vi "NIIE_MouseDown.vi"(7 "Flip Colors?":bool, 8 "Error":errorcluster, 10 "Coords":T5, 11 "Data":T1={"Class"={"Ants"=refnum, "Layer"=refnum, "Templates"=refnum, "Icon"=refnum, "Glyph"=refnum, "Settings"=refnum, "Tools"=refnum}, "Ref"={"Add Layer"=refnum, "Remove Layer"=refnum, "Line Text"=[], "Body Text Spec"=refnum, "DNL_Font"=refnum, "glyph path str"=refnum, "templates path str"=refnum, "Arrow Up"=refnum, "Arrow Down"=refnum, "IE VI Ref"=refnum, "Glyphs tree"=refnum, "Templates tree"=refnum, "Layer Icon Text"=refnum, "Layer Template"=refnum, "Clipboard"=refnum, "BW icon in"=refnum, "Color icon in"=refnum, "Layer Clust"=refnum, "Body Text"=refnum, "DNL_Framework Templates"=refnum, "Search Templates"=refnum, "TextMarker"=refnum, "Tab Control"=refnum, "Search Glyphs"=refnum, "Line Color"=refnum, "DNL_Glyphs []"=refnum, "Fill Color"=refnum, "Tools"=refnum, "Glyphs tree"=refnum, "Icon"=refnum, "Preview"=refnum, "Ants"=refnum, "Terminals"=refnum, "menu reference"=refnum, "LayerNames"=[], "GlyphLoadAnimation"=refnum, "TemplateLoadAnimation"=refnum, "refreshGlyphs"=refnum, "refreshTemplates"=refnum}, "Support"={"AntsRect"={"left"=0, "top"=0, "right"=0, "bottom"=0}, "Mouse Move Coords"={"Horizontal"=0, "Vertical"=0}, "Mouse Down Coords"={"Horizontal"=0, "Vertical"=0}, "Temp Coord"={"Horizontal"=0, "Vertical"=0}, "Action"=enum."Default", "Edge Color"=4914962, "Fill Color"=16860, "Mouse Down?"=FALSE, "Draft Mode?"=FALSE, "Temp Icon"=bytes[3102], "CTRL Pressed"=FALSE, "Move Selection?"=FALSE, "AntsRect Orig"={"left"=0, "top"=0, "right"=0, "bottom"=0}, "Text"="", "TM Set?"=FALSE, "Mouse inside icon?"=FALSE, "Tool (old value)"=0, "Pencil Move Color"=0, "Swap Colors?"=FALSE, "Shift pressed?"=FALSE}}) -> (0 "Error Out":errorcluster, 3 "Data Out":T1={"Class"={"Ants"=refnum, "Layer"=refnum, "Templates"=refnum, "Icon"=refnum, "Glyph"=refnum, "Settings"=refnum, "Tools"=refnum}, "Ref"={"Add Layer"=refnum, "Remove Layer"=refnum, "Line Text"=[], "Body Text Spec"=refnum, "DNL_Font"=refnum, "glyph path str"=refnum, "templates path str"=refnum, "Arrow Up"=refnum, "Arrow Down"=refnum, "IE VI Ref"=refnum, "Glyphs tree"=refnum, "Templates tree"=refnum, "Layer Icon Text"=refnum, "Layer Template"=refnum, "Clipboard"=refnum, "BW icon in"=refnum, "Color icon in"=refnum, "Layer Clust"=refnum, "Body Text"=refnum, "DNL_Framework Templates"=refnum, "Search Templates"=refnum, "TextMarker"=refnum, "Tab Control"=refnum, "Search Glyphs"=refnum, "Line Color"=refnum, "DNL_Glyphs []"=refnum, "Fill Color"=refnum, "Tools"=refnum, "Glyphs tree"=refnum, "Icon"=refnum, "Preview"=refnum, "Ants"=refnum, "Terminals"=refnum, "menu reference"=refnum, "LayerNames"=[], "GlyphLoadAnimation"=refnum, "TemplateLoadAnimation"=refnum, "refreshGlyphs"=refnum, "refreshTemplates"=refnum}, "Support"={"AntsRect"={"left"=0, "top"=0, "right"=0, "bottom"=0}, "Mouse Move Coords"={"Horizontal"=0, "Vertical"=0}, "Mouse Down Coords"={"Horizontal"=0, "Vertical"=0}, "Temp Coord"={"Horizontal"=0, "Vertical"=0}, "Action"=enum."Default", "Edge Color"=4914962, "Fill Color"=16860, "Mouse Down?"=FALSE, "Draft Mode?"=FALSE, "Temp Icon"=bytes[3102], "CTRL Pressed"=FALSE, "Move Selection?"=FALSE, "AntsRect Orig"={"left"=0, "top"=0, "right"=0, "bottom"=0}, "Text"="", "TM Set?"=FALSE, "Mouse inside icon?"=FALSE, "Tool (old value)"=0, "Pencil Move Color"=0, "Swap Colors?"=FALSE, "Shift pressed?"=FALSE}})   [LabVIEW 2021]
uses:
  <vilib>/Utility/miscctls.llb/LVPoint32TypeDef.ctl
  Controls/IE Data.ctl
  Class/Ants/Ants.lvclass
  Class/FakedArray/FakedArray.lvclass
  Class/Icon Library/Glyph.lvclass
  Class/Settings/Settings.lvclass
  Class/Tools/Tools Paint.lvclass
  vi.lib/LabVIEW Icon API/lv_icon/Classes/Icon/Icon.lvclass
  Controls/IE Classes.ctl
  Controls/References Cluster.ctl
  Controls/SupportClass.ctl
  Controls/ENUM_SupportClass_Action.ctl
  vi.lib/LabVIEW Icon API/lv_icon/Controls/IEColor.ctl
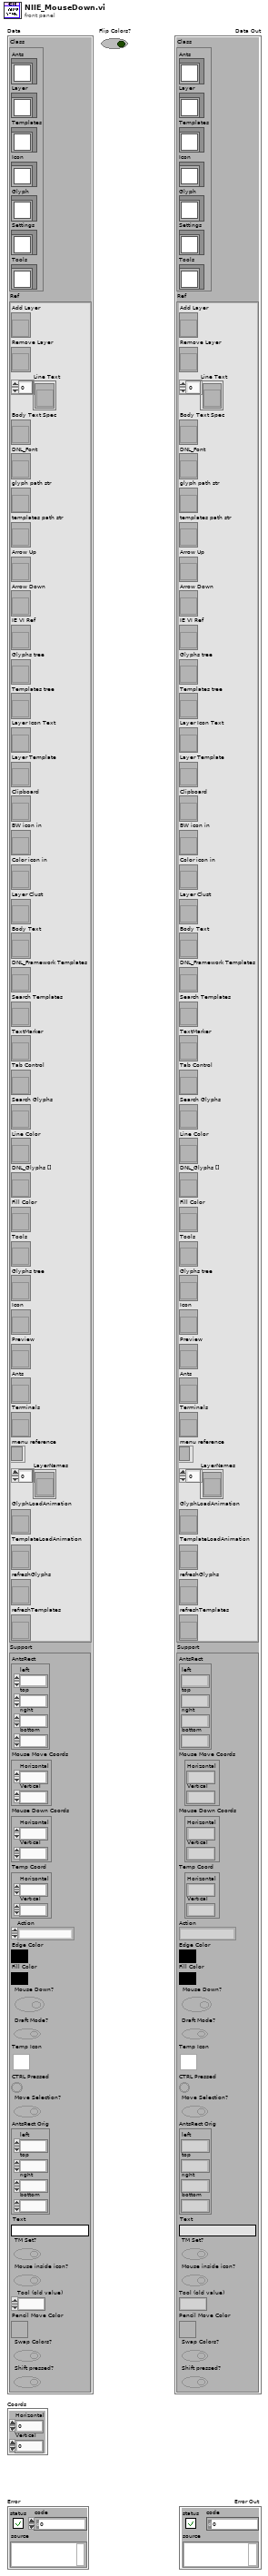
[diagram p1: front panel]
types:
  T1 = typedef "IE Data.ctl" = cluster{"Class":T2, "Ref":T3, "Support":T4}
  T2 = typedef "IE Classes.ctl" = cluster{"Ants":refnum<class "Ants.lvclass">, "Layer":refnum<class "FakedArray.lvclass">, "Templates":refnum<class "FakedArray.lvclass">, "Icon":refnum<class "Icon.lvclass">, "Glyph":refnum<class "Glyph.lvclass">, "Settings":refnum<class "Settings.lvclass">, "Tools":refnum<class "Tools Paint.lvclass">}
  T3 = typedef "References Cluster.ctl" = cluster{"Add Layer":refnum<vi>, "Remove Layer":refnum<vi>, "Line Text":refnum<vi>[], "Body Text Spec":refnum<vi>, "DNL_Font":refnum<vi>, "glyph path str":refnum<vi>, "templates path str":refnum<vi>, "Arrow Up":refnum<vi>, "Arrow Down":refnum<vi>, "IE VI Ref":refnum<vi>, "Glyphs tree":refnum<vi>, "Templates tree":refnum<vi>, "Layer Icon Text":refnum<vi>, "Layer Template":refnum<vi>, "Clipboard":refnum<vi>, "BW icon in":refnum<vi>, "Color icon in":refnum<vi>, "Layer Clust":refnum<vi>, "Body Text":refnum<vi>, "DNL_Framework Templates":refnum<vi>, "Search Templates":refnum<vi>, "TextMarker":refnum<vi>, "Tab Control":refnum<vi>, "Search Glyphs":refnum<vi>, "Line Color":refnum<vi>, "DNL_Glyphs []":refnum<vi>, "Fill Color":refnum<vi>, "Tools":refnum<vi>, "Glyphs tree":refnum<vi>, "Icon":refnum<vi>, "Preview":refnum<vi>, "Ants":refnum<vi>, "Terminals":refnum<vi>, "menu reference":refnum<k9>, "LayerNames":refnum<vi>[], "GlyphLoadAnimation":refnum<vi>, "TemplateLoadAnimation":refnum<vi>, "refreshGlyphs":refnum<vi>, "refreshTemplates":refnum<vi>}
  T4 = typedef "SupportClass.ctl" = cluster{"AntsRect":cluster{"left":i16, "top":i16, "right":i16, "bottom":i16}, "Mouse Move Coords":T5, "Mouse Down Coords":T5, "Temp Coord":T5, "Action":T6, "Edge Color":T7, "Fill Color":T7, "Mouse Down?":bool, "Draft Mode?":bool, "Temp Icon":picture, "CTRL Pressed":bool, "Move Selection?":bool, "AntsRect Orig":cluster{"left":i16, "top":i16, "right":i16, "bottom":i16}, "Text":string, "TM Set?":bool, "Mouse inside icon?":bool, "Tool (old value)":u32, "Pencil Move Color":u32, "Swap Colors?":bool, "Shift pressed?":bool}
  T5 = typedef "LVPoint32TypeDef.ctl" = cluster{"Horizontal":i32, "Vertical":i32}
  T6 = typedef "ENUM_SupportClass_Action.ctl" = enum16{"Default", "Move Selection", "Glyph Library", "Tool"}
  T7 = typedef "IEColor.ctl" = u32
  T8 = cluster{"left":i16, "top":i16, "right":i16, "bottom":i16}
  T9 = typedef "Cluster_Button Draw Tools.ctl" = enum32{"Pencil", "Line", "Dropper", "Fill", "Rectangle", "Filled Rectangle", "Ellipse", "Filled Ellipse", "Eraser", "Text", "Select", "Move"}
  T10 = cluster{"Horizontal":i32, "Vertical":i32, "Vertical 2":i32, "Vertical 3":i32}
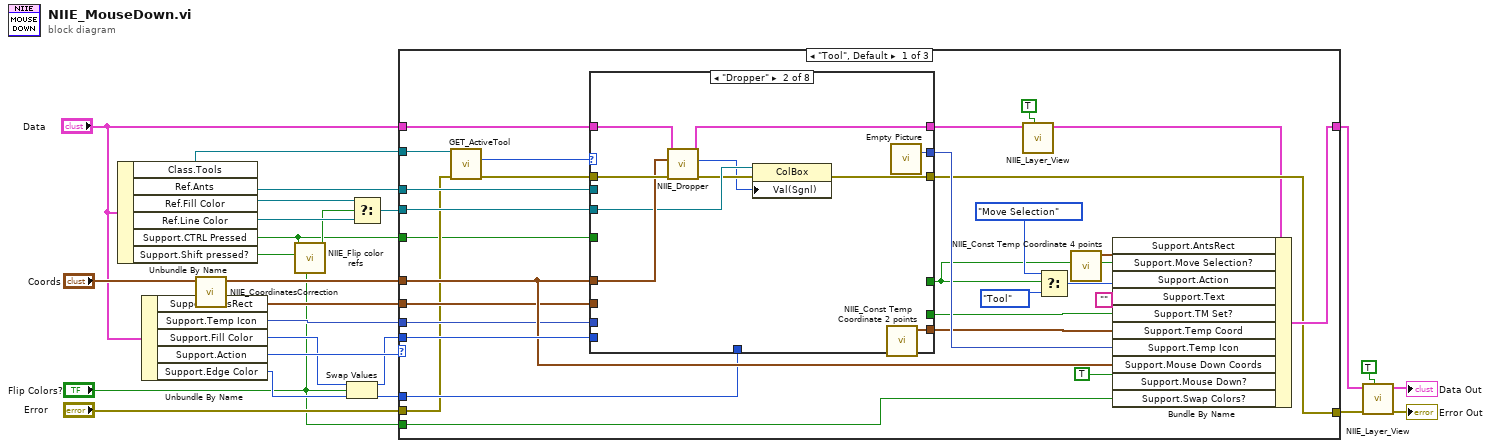
[diagram p0: block diagram]
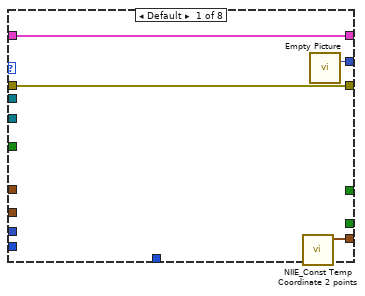
[diagram p2: hidden frame]
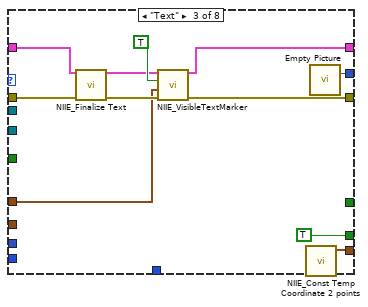
[diagram p3: hidden frame]
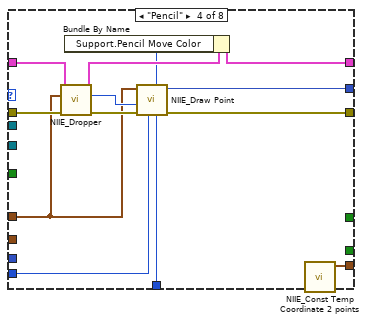
[diagram p4: hidden frame]
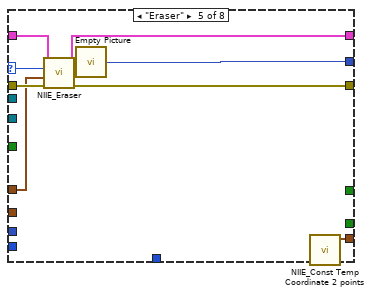
[diagram p5: hidden frame]
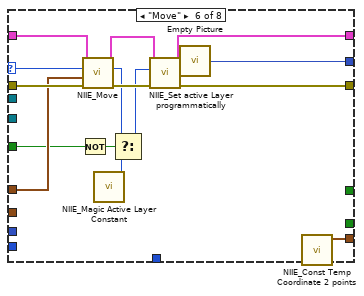
[diagram p6: hidden frame]
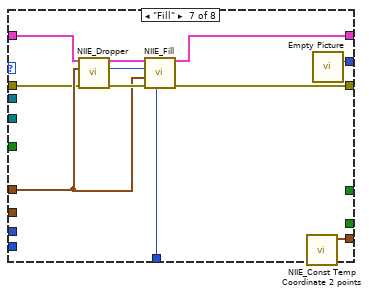
[diagram p7: hidden frame]
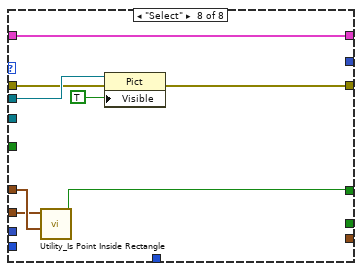
[diagram p8: hidden frame]
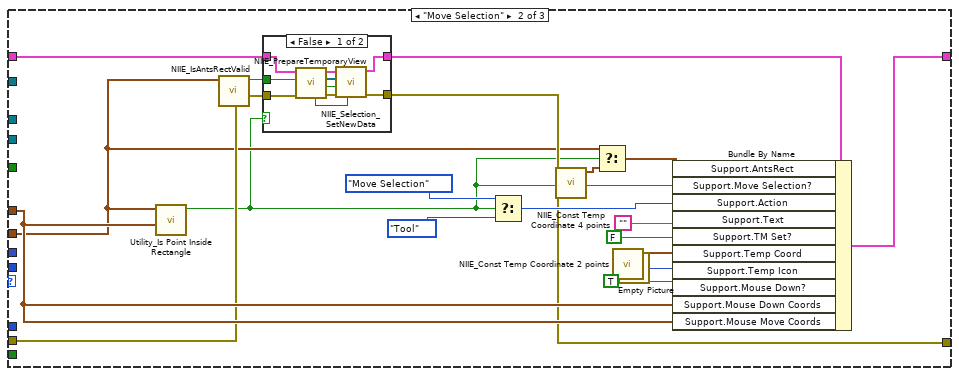
[diagram p9: hidden frame]
diagram:
  n1 = Unbundle By Name("Data") -> ("Class.Tools"=w19:refnum<class "Tools Paint.lvclass">, "Ref.Ants"=w21:refnum<vi>, "Ref.Fill Color"=w6:refnum<vi>, "Ref.Line Color"=w5:refnum<vi>, "Support.CTRL Pressed"=w1:bool, "Support.Shift pressed?"=w2:bool)
  n2 = Unbundle By Name("Data") -> ("Support.AntsRect"=w20:T8, "Support.Temp Icon"=w22:picture, "Support.Fill Color"=w9:T7, "Support.Action"=w24:T6, "Support.Edge Color"=w11:T7)
  n3 = call "NIIE_CoordinatesCorrection.vi"("Coordinates In"="Coords") -> ("Corrected Out"=w25:T5)  [unwired: 10 out]
  n4 = call "NIIE_Flip color refs.vi"("Flip colors?"="Flip Colors?", "Shift pressed"=w2, "CTRL pressed"=w1) -> ("Flip?"=w3:bool)  [unwired: 8 out]
  n5 = Swap Values(12:w9, 13:"Flip Colors?", 14:w11) -> (1:w8:T7, 3:w10:T7)
  n6 = Select(t=w6, s=w3, f=w5) -> (s? t:f=w7:refnum<vi>)
  n7 = case shown="\"Tool\", Default" w24 {
    tunnel: [w47 w141 w167] -> w15
    tunnel: w25 -> [w50 w144 _]
    tunnel: "Error" -> [w34 w142 w167]
    tunnel: [w48 w149 w166] -> w12
    tunnel: w8 -> [w51 _ _]
    tunnel: w10 -> [w46 _ _]
    tunnel: w22 -> [w43 _ _]
    tunnel: w21 -> [w42 _ _]
    tunnel: w20 -> [w41 w138 _]
    tunnel: w7 -> [w37 _ _]
    tunnel: w19 -> [w35 _ _]
    tunnel: "Data" -> [w33 w140 w166]
    tunnel: "Flip Colors?" -> [w32 _ _]
    tunnel: w1 -> [w30 _ _]
    frame "Tool", Default {
      n8 = call-dynamic "GET_ActiveTool.vi"("error in (no error)"=w34, "Tools Paint.lvclass in"=w35) -> ("error out"=w53:errorcluster, "Radio Buttons"=w54:T9)  [unwired: 8 out]
      n9 = case shown="\"Dropper\"" w54 {
        selector: w54 -> [_ _ _ _ w96 w112 _ _]
        tunnel: w53 -> [w58 w67 w75 w90 w99 w114 w121 w129]
        tunnel: w50 -> [_ w65 w69 w81 w97 w113 w122 w131]
        tunnel: w51 -> [_ _ _ w82 _ _ _ _]
        tunnel: [w57 w68 w76 w80 w100 w115 w125 _] -> w49
        tunnel: [w58 w66 w78 w92 w98 w109 w124 w132] -> w47
        tunnel: w46 -> [_ _ _ w83 _ _ w116 _]
        tunnel: [w56 w64 w79 w91 w95 w111 w126 _] -> w45
        tunnel: [_ _ TRUE ("Mouse Down?") _ _ _ _ _] -> w44
        tunnel: w43 -> [_ _ _ _ _ _ _ _]
        tunnel: w42 -> [_ _ _ _ _ _ _ w134]
        tunnel: w41 -> [_ _ _ _ _ _ _ w130]
        tunnel: [_ _ _ _ _ _ _ w127] -> w36
        tunnel: w37 -> [_ w63 _ _ _ _ _ _]
        tunnel: w33 -> [w55 w62 w73 w87 w94 w108 w119 w128]
        tunnel: [w55 w61 w70 w85 w93 w106 w117 w128] -> w28
        tunnel: w30 -> [_ _ _ _ _ w105 _ _]
        frame Default {
          n10 = call "NIIE_Const Temp Coordinate 2 points.vi"() -> ("Const Temp Coordinate"=w56:T5)  [unwired: 11 out]
          n11 = call "Empty Picture"() -> ("empty picture"=w57:picture)
        }
        frame "Dropper" {
          n12 = call "NIIE_Dropper.vi"("Error"=w67, "Point"=w65, "Data"=w62) -> ("Error Out"=w60:errorcluster, "Color Out"=w59:u32, "Data Out"=w61:T1)  [unwired: 1 in, 5 out]
          n13 = property on="Property Node" class="ColBox"(reference=w63, error in=w60, "Val(Sgnl)"=w59) -> (error out=w66:errorcluster)  [unwired: 1 out]
          n14 = call "NIIE_Const Temp Coordinate 2 points.vi"() -> ("Const Temp Coordinate"=w64:T5)  [unwired: 11 out]
          n15 = call "Empty Picture"() -> ("empty picture"=w68:picture)
        }
        frame "Text" {
          n16 = call "NIIE_Finalize Text.vi"("Error"=w75, "Data"=w73) -> ("Error Out"=w74:errorcluster, "Data Out"=w71:T1)  [unwired: 8 out]
          n17 = call "NIIE_VisibleTextMarker.vi"("Error"=w74, "Positon"=w69, "Visible"=TRUE, "Data"=w71) -> ("Error Out"=w78:errorcluster, "Data Out"=w70:T1)  [unwired: 6 out]
          n18 = call "NIIE_Const Temp Coordinate 2 points.vi"() -> ("Const Temp Coordinate"=w79:T5)  [unwired: 11 out]
          n19 = call "Empty Picture"() -> ("empty picture"=w76:picture)
        }
        frame "Pencil" {
          n20 = call "NIIE_Dropper.vi"("Error"=w90, "Point"=w81, "Data"=w87) -> ("Error Out"=w89:errorcluster, "Color Out"=w88:u32, "Data Out"=w86:T1)  [unwired: 6 out]
          n21 = call "NIIE_Draw Point.vi"("Edge Color"=w83, "Fill Color"=w82, "Error"=w89, "Current Color (T)"=w88, "Point(x,y)"=w81) -> ("Error Out"=w92:errorcluster, "New Picture Out"=w80:picture, "Current Line Color Out"=w84:u32)  [unwired: 4 in]
          n22 = Bundle By Name(cluster=w86, "Support.Pencil Move Color"=w84) -> (w85:T1)
          n23 = call "NIIE_Const Temp Coordinate 2 points.vi"() -> ("Const Temp Coordinate"=w91:T5)  [unwired: 11 out]
        }
        frame "Eraser" {
          n24 = call "NIIE_Eraser.vi"("Error"=w99, "Point Out"=w97, "Radio Buttons"=w96, "Data"=w94) -> ("Error Out"=w98:errorcluster, "Data Out"=w93:T1)  [unwired: 1 in, 5 out]
          n25 = call "Empty Picture"() -> ("empty picture"=w100:picture)
          n26 = call "NIIE_Const Temp Coordinate 2 points.vi"() -> ("Const Temp Coordinate"=w95:T5)  [unwired: 11 out]
        }
        frame "Move" {
          n27 = Not(x=w105) -> (.not. x?=w104:bool)
          n28 = call "NIIE_Move.vi"("Error"=w114, "Point(x,y)"=w113, "Tools"=w112, "Data"=w108) -> ("Error Out"=w110:errorcluster, "Active Layer Out"=w103:i32, "Data Out"=w107:T1)  [unwired: 1 in, 4 out]
          n29 = call "NIIE_Magic Active Layer Constant.vi"() -> ("Magic Constant"=w102:i32)  [unwired: 11 in]
          n30 = Select(t=w103, s=w104, f=w102) -> (s? t:f=w101:i32)
          n31 = call "NIIE_Set active Layer programmatically.vi"("Error"=w110, "Active Layer"=w101, "Data"=w107) -> ("Error Out"=w109:errorcluster, "Data Out"=w106:T1)  [unwired: 1 in, 6 out]
          n32 = call "Empty Picture"() -> ("empty picture"=w115:picture)
          n33 = call "NIIE_Const Temp Coordinate 2 points.vi"() -> ("Const Temp Coordinate"=w111:T5)  [unwired: 11 out]
        }
        frame "Fill" {
          n34 = call "NIIE_Dropper.vi"("Error"=w121, "Point"=w122, "Data"=w119) -> ("Error Out"=w123:errorcluster, "Color Out"=w120:u32, "Data Out"=w118:T1)  [unwired: 6 out]
          n35 = call "NIIE_Fill.vi"("Color"=w116, "Error"=w123, "Point"=w122, "Ref Color"=w120, "Data"=w118) -> ("Error Out"=w124:errorcluster, "Data Out"=w117:T1)  [unwired: 1 in, 4 out]
          n36 = call "NIIE_Const Temp Coordinate 2 points.vi"() -> ("Const Temp Coordinate"=w126:T5)  [unwired: 11 out]
          n37 = call "Empty Picture"() -> ("empty picture"=w125:picture)
        }
        frame "Select" {
          n38 = call "Utility_Is Point Inside Rectangle.vi"("Point"=w131, "Rectangle"=w130) -> ("Inside? Out"=w127:bool)  [unwired: 9 out]
          n39 = property class="Pict"(reference=w134, error in=w129, "Visible"=TRUE) -> (error out=w132:errorcluster)  [unwired: 1 out]
        }
      }
      n40 = call "NIIE_Layer_View.vi"("Add To Undo?"=TRUE ("Add to Undo?"), "Data"=w28) -> ("Data Out"=w27:T1)  [unwired: 2 in, 7 out]
      n41 = Select(t=ENUM_SupportClass_Action."Move Selection", s=w36, f=ENUM_SupportClass_Action."Tool" ("Action")) -> (s? t:f=w38:T6)
      n42 = call "NIIE_Const Temp Coordinate 4 points.vi"() -> ("Const Temp Coordinate"=w31:T10)  [unwired: 11 out]
      n43 = Bundle By Name(cluster=w27, "Support.AntsRect"=w31, "Support.Move Selection?"=w36, "Support.Action"=w38, "Support.Text"="", "Support.TM Set?"=w44, "Support.Temp Coord"=w45, "Support.Temp Icon"=w49, "Support.Mouse Down Coords"=w50, "Support.Mouse Down?"=TRUE ("Mouse Down?"), "Support.Swap Colors?"=w32) -> (w48:T1)
    }
    frame "Move Selection" {
      n44 = call "Utility_Is Point Inside Rectangle.vi"("Point"=w144, "Rectangle"=w138) -> ("Inside? Out"=w135:bool)  [unwired: 9 out]
      n45 = call "NIIE_IsAntsRectValid.vi"("Image Range"=w138) -> ("Valid? Out"=w143:bool)  [unwired: 10 out]
      n46 = case shown="False" w135 {
        tunnel: w143 -> [w160 _]
        tunnel: w142 -> [w159 w165]
        tunnel: [w158 w165] -> w141
        tunnel: w140 -> [w156 w164]
        tunnel: [w154 w164] -> w139
        frame False {
          n47 = call "NIIE_PrepareTemporaryView.vi"("Error"=w159, "Valid Selection?"=w160, "Data"=w156) -> ("Error Out"=w157:errorcluster, "Highlighted? Out"=w162:bool, "All Layers Out"=w163:refnum<class "Layer.lvclass">[], "Data Out"=w155:T1, "#Active Layer Out"=w161:i32)  [unwired: 2 in, 2 out]
          n48 = call "NIIE_Selection_SetNewData.vi"("#Active Layer"=w161, "Error"=w157, "Highlighted?"=w162, "All Layers"=w163, "Data"=w155) -> ("Error Out"=w158:errorcluster, "Data Out"=w154:T1)  [unwired: 1 in, 3 out]
        }
        frame True {
        }
      }
      n49 = Select(t=ENUM_SupportClass_Action."Move Selection", s=w135, f=ENUM_SupportClass_Action."Tool") -> (s? t:f=w148:T6)
      n50 = call "NIIE_Const Temp Coordinate 4 points.vi"() -> ("Const Temp Coordinate"=w137:T10)  [unwired: 11 out]
      n51 = Select(t=w138, s=w135, f=w137) -> (s? t:f=w136:T10)
      n52 = call "NIIE_Const Temp Coordinate 2 points.vi"() -> ("Const Temp Coordinate"=w147:T5)  [unwired: 11 out]
      n53 = call "Empty Picture"() -> ("empty picture"=w146:picture)
      n54 = Bundle By Name(cluster=w139, "Support.AntsRect"=w136, "Support.Move Selection?"=w135, "Support.Action"=w148, "Support.Text"="", "Support.TM Set?"=FALSE ("TM Set?"), "Support.Temp Coord"=w147, "Support.Temp Icon"=w146, "Support.Mouse Down?"=TRUE ("Mouse Down?"), "Support.Mouse Down Coords"=w144, "Support.Mouse Move Coords"=w144) -> (w149:T1)
    }
    frame "Glyph Library" {
    }
  }
  n55 = call "NIIE_Layer_View.vi"("Add To Undo?"=TRUE ("Add to Undo?"), "Error"=w15, "Data"=w12) -> ("Error Out"=→"Error Out":errorcluster, "Data Out"=→"Data Out":T1)  [unwired: 1 in, 6 out]
